vi "SampleApplication.vi"() -> ()   [LabVIEW 2009]
uses:
  TofDaqDll/TSharedMemoryDesc.ctl
  TofDaqDll/Dblx16.ctl
  TofDaqDll/charX256.ctl
  TofDaqDll/charX128.ctl
panel:
  in  "TSharedMemoryDesc":T1
  out "TofDaq running":bool
  out "peak mass":sgl
  out "peak label":string
  in  "peak index":i32
  out "profile":T5(graph)
  out "Mass Spec Axis Label":string
  in  "stop":bool
  in  "Stop":bool
  in  "Start":bool
  out "DAQ active":bool
  out "Mass spectra":T6(graph)
  in  "Axis type":i32=1
  in  "Normalize":bool=TRUE
  in  "SegmentIndex":i32 min=0 max=9 step=1
  out "error out":errorcluster
  in  "error in (no error)":errorcluster
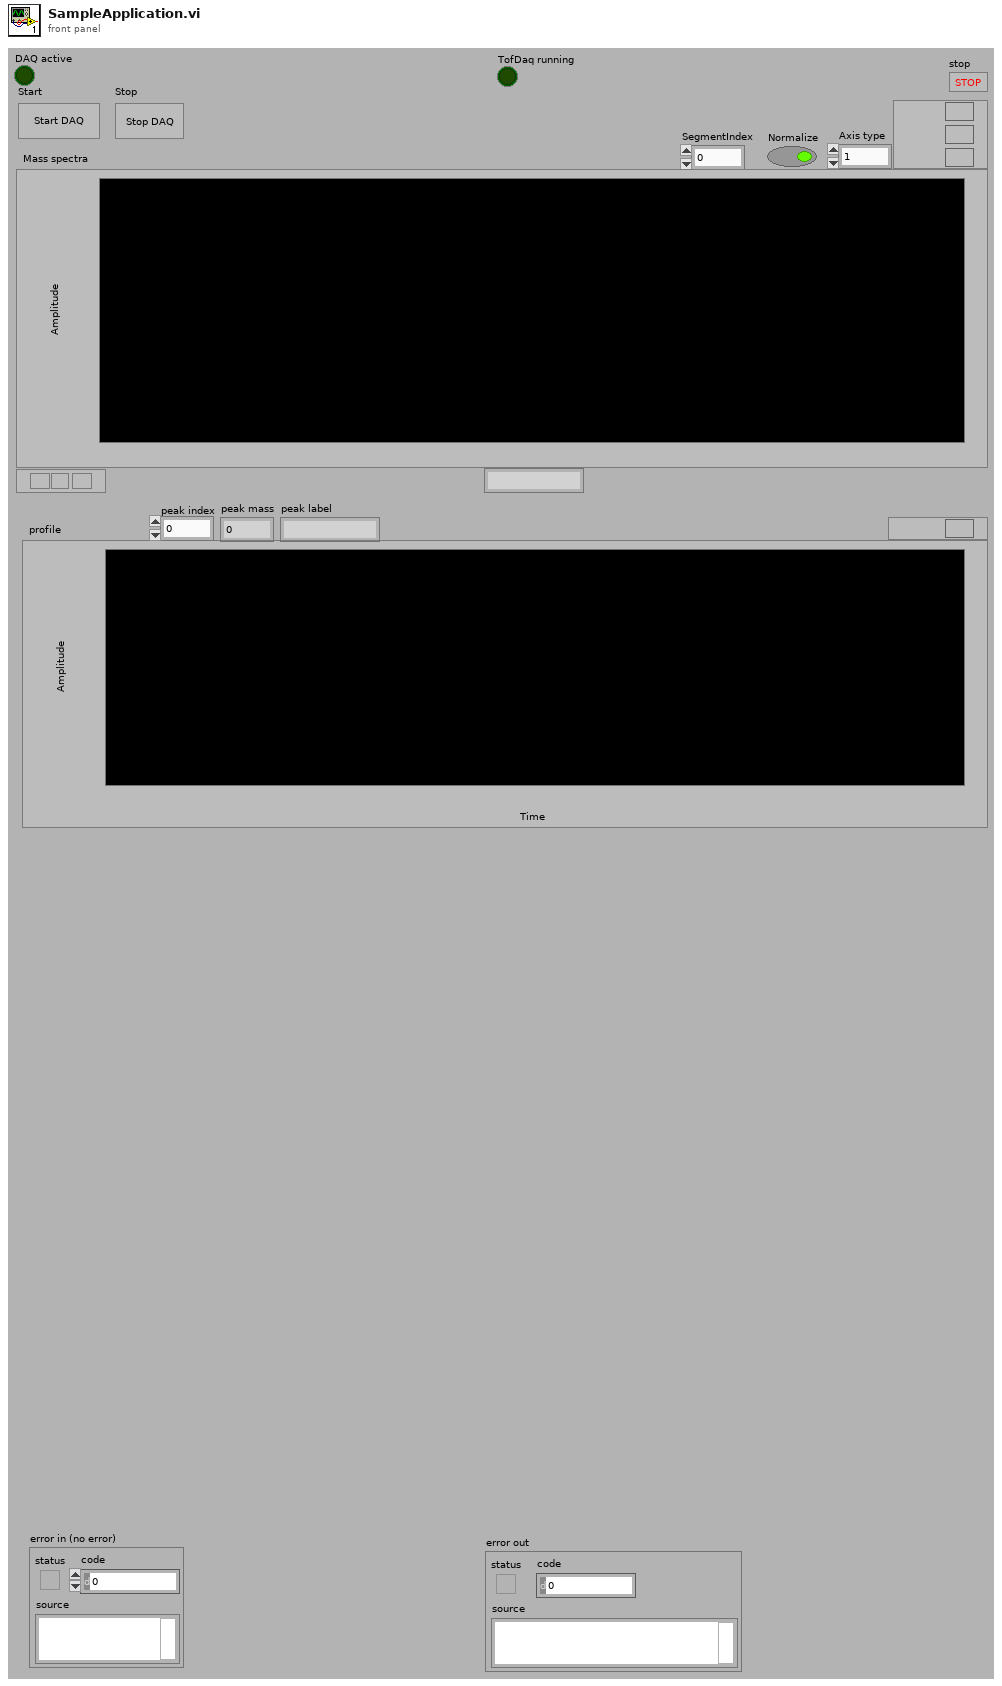
[diagram p1: front panel]
types:
  T1 = typedef "TSharedMemoryDesc.ctl" = cluster{"NbrSamples":i32, "NbrRawSamples":i32, "NbrPeaks":i32, "NbrWaveforms":i32, "NbrSegments":i32, "NbrBlocks":i32, "NbrMemories":i32, "NbrBufs":i32, "NbrWrites":i32, "NbrRuns":i32, "iWaveform":i32, "iSegment":i32, "iBlock":i32, "iMemory":i32, "iBuf":i32, "iWrite":i32, "iRun":i32, "TotalBufsRecorded":i32, "TotalBufsProcessed":i32, "TotalBufsWritten":i32, "OverallBufsProcessed":i32, "TotalNbrMemories":i32, "TotalMemoriesProcessed":i32, "RawDataRecordedBuf1":u32, "RawDataRecordedBuf2":u32, " RawDataLastElementInBuffer1 ":u32, " RawDataLastElementInBuffer2":u32, "RawDataProcessedBuf1":u32, "RawDataProcessedBuf2":u32, "RawDataWrittenBuf1":u32, "RawDataWrittenBuf2":u32, "SampleInterval":sgl, "TofPeriod":i32, "dummy":i32, "BlockPeriod":i64, "BlockPulseDelay":i64, " BlockDelay ":i64, "SingleIonSignal":sgl, "SingleIonSignal2":sgl, "MassCalibMode":i32, "MassCalibMode2":i32, "NbrMassCalibParams":i32, "NbrMassCalibParams2":i32, "p":T2, "p2":T2, "R0":sgl, "dm":sgl, "m0":sgl, "secondTof":u8, "chIniFileName":T3, "CurrentDataFileName":T3, "dummy":i8, "dummy 2":i8, "dummy 3":i8, "DaqMode":i32, " AcquisitionMode ":i32, "CombineMode":i32, "RecalibFreq":i32, "AcquisitionLogText":T3, " AcquisitionLogTime ":u64, "TimeZero":u64, "ExternalLock":u32, "ProcessingLevel":u32, "AttributeType":i32, "AttributeObject":T3, "AttributeName":T4, " AttributeInt ":i32, " AttributeDouble ":dbl, "EnableVarNbrMemories":u8, "dummy 4":i8, "dummy 5":i8, "dummy 6":i8, " NbrSteps":i32, "  CurrentStepAtBuf ":i32, "NbrMemoriesForCurrentStep":i32}
  T2 = typedef "Dblx16.ctl" = cluster{"0":dbl, "1":dbl, "2":dbl, "3":dbl, "4":dbl, "5":dbl, "6":dbl, "7":dbl, "8":dbl, "9":dbl, "10":dbl, "11":dbl, "12":dbl, "13":dbl, "14":dbl, "15":dbl}
  T3 = typedef "charX256.ctl" = cluster{i8, i8, i8, i8, i8, i8, i8, i8, i8, i8, i8, i8, i8, i8, i8, i8, i8, i8, i8, i8, i8, i8, i8, i8, i8, i8, i8, i8, i8, i8, i8, i8, i8, i8, i8, i8, i8, i8, i8, i8, i8, i8, i8, i8, i8, i8, i8, i8, i8, i8, i8, i8, i8, i8, i8, i8, i8, i8, i8, i8, i8, i8, i8, i8, i8, i8, i8, i8, i8, i8, i8, i8, i8, i8, i8, i8, i8, i8, i8, i8, i8, i8, i8, i8, i8, i8, i8, i8, i8, i8, i8, i8, i8, i8, i8, i8, i8, i8, i8, i8, i8, i8, i8, i8, i8, i8, i8, i8, i8, i8, i8, i8, i8, i8, i8, i8, i8, i8, i8, i8, i8, i8, i8, i8, i8, i8, i8, i8, i8, i8, i8, i8, i8, i8, i8, i8, i8, i8, i8, i8, i8, i8, i8, i8, i8, i8, i8, i8, i8, i8, i8, i8, i8, i8, i8, i8, i8, i8, i8, i8, i8, i8, i8, i8, i8, i8, i8, i8, i8, i8, i8, i8, i8, i8, i8, i8, i8, i8, i8, i8, i8, i8, i8, i8, i8, i8, i8, i8, i8, i8, i8, i8, i8, i8, i8, i8, i8, i8, i8, i8, i8, i8, i8, i8, i8, i8, i8, i8, i8, i8, i8, i8, i8, i8, i8, i8, i8, i8, i8, i8, i8, i8, i8, i8, i8, i8, i8, i8, i8, i8, i8, i8, i8, i8, i8, i8, i8, i8, i8, i8, i8, i8, i8, i8, i8, i8, i8, i8, i8, i8, i8, i8, i8, i8, i8, i8}
  T4 = typedef "charX128.ctl" = cluster{i8, i8, i8, i8, i8, i8, i8, i8, i8, i8, i8, i8, i8, i8, i8, i8, i8, i8, i8, i8, i8, i8, i8, i8, i8, i8, i8, i8, i8, i8, i8, i8, i8, i8, i8, i8, i8, i8, i8, i8, i8, i8, i8, i8, i8, i8, i8, i8, i8, i8, i8, i8, i8, i8, i8, i8, i8, i8, i8, i8, i8, i8, i8, i8, i8, i8, i8, i8, i8, i8, i8, i8, i8, i8, i8, i8, i8, i8, i8, i8, i8, i8, i8, i8, i8, i8, i8, i8, i8, i8, i8, i8, i8, i8, i8, i8, i8, i8, i8, i8, i8, i8, i8, i8, i8, i8, i8, i8, i8, i8, i8, i8, i8, i8, i8, i8, i8, i8, i8, i8, i8, i8, i8, i8, i8, i8, i8, i8}
  T5 = cluster{"profile time":dbl[], "profile data":sgl[]}
  T6 = cluster{"SpecAxis out":dbl[], "SumSpectrum out":dbl[]}[]
  T7 = cluster{"label":string, "mass":sgl, "loMass":sgl, "hiMass":sgl}
  T8 = cluster{"SpecAxis out":dbl[], "Tof spectrum out":sgl[]}
  T9 = cluster{"Masses out":sgl[], "Stick spectrum out":sgl[]}
  T10 = cluster{"SpecAxis out":dbl[], "SumSpectrum out":dbl[]}
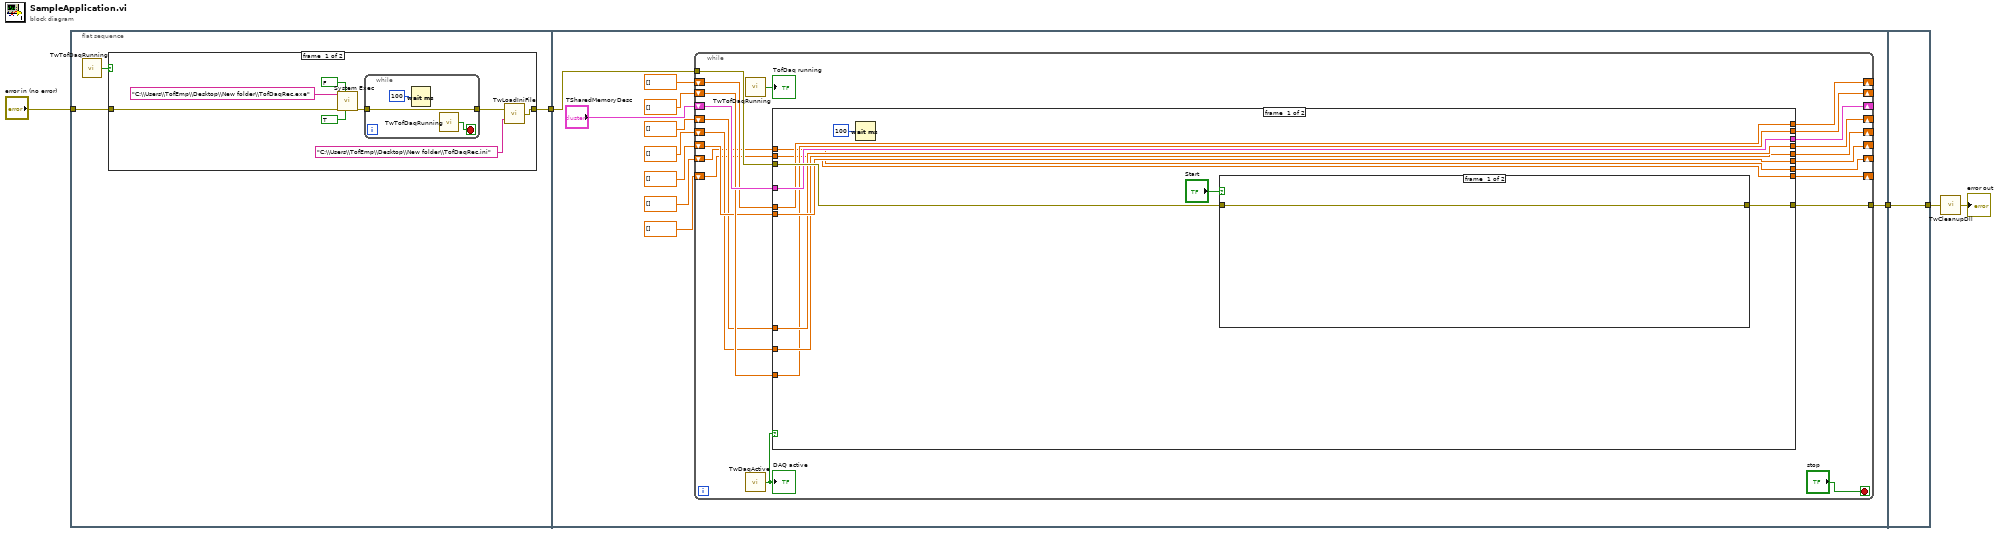
[diagram p0: block diagram]
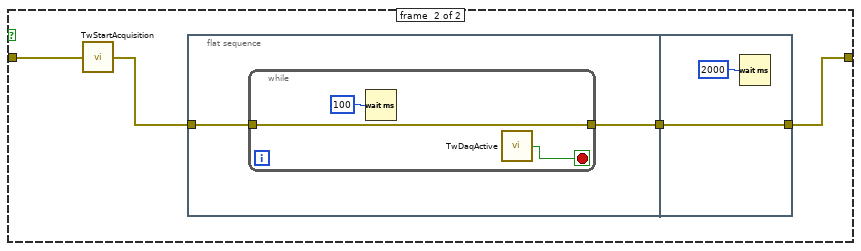
[diagram p3: hidden frame]
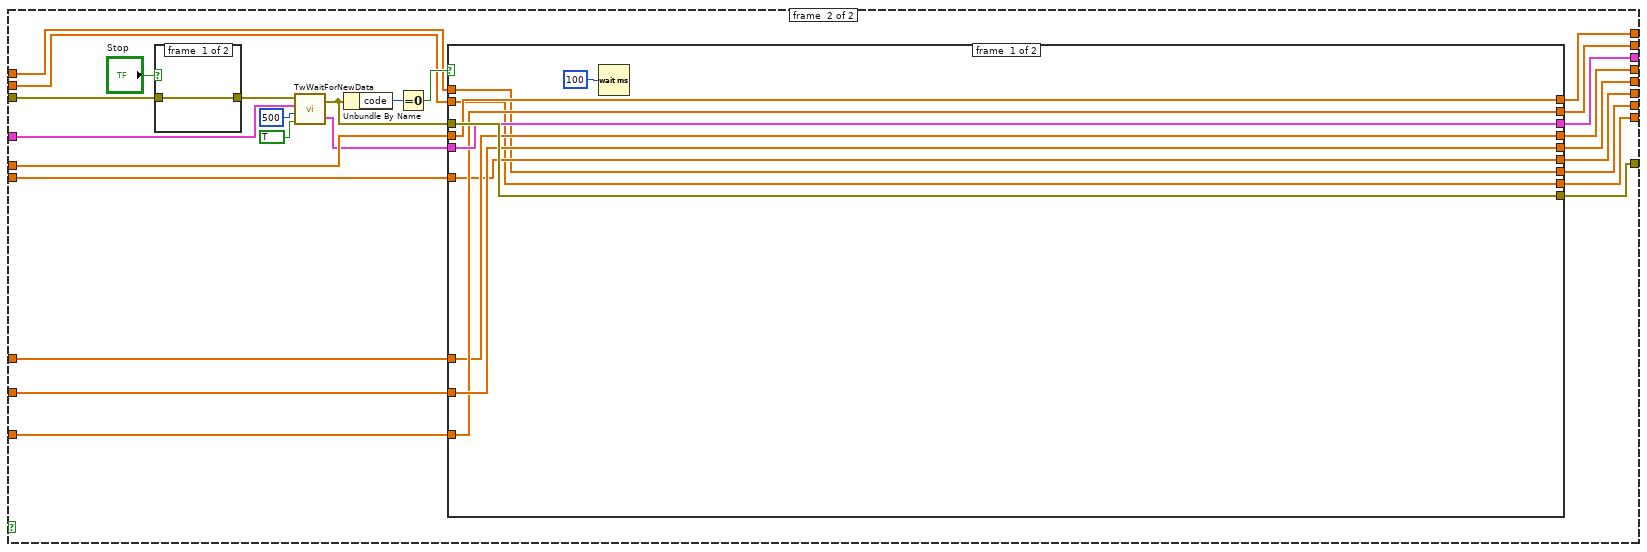
[diagram p4: hidden frame]
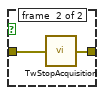
[diagram p5: hidden frame]
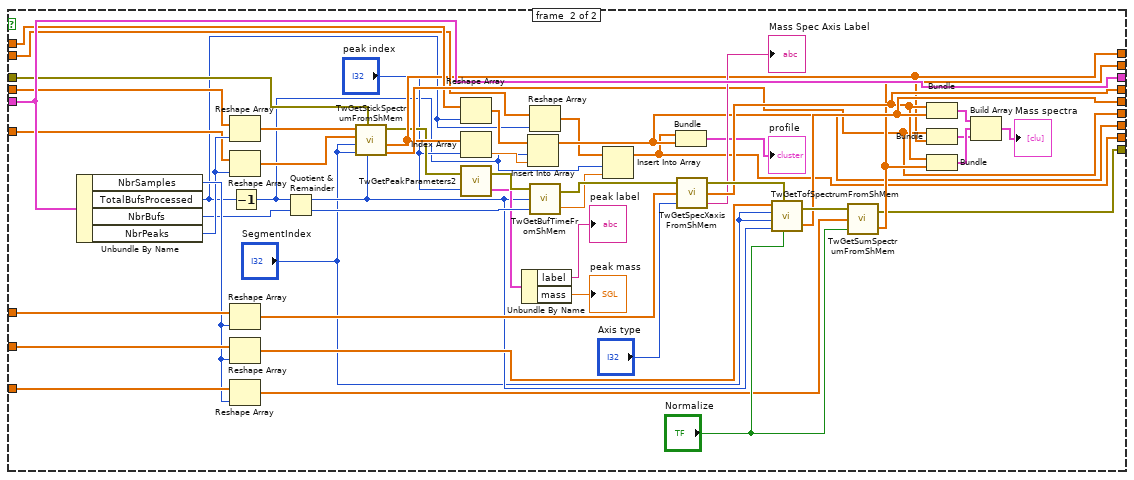
[diagram p6: hidden frame]
diagram:
  n1 = flat-sequence {
    tunnel: "error in (no error)" -> [w7]
    tunnel: [w6] -> w5
    tunnel: w5 -> [w30]
    tunnel: [w22] -> w4
    tunnel: [w166] -> w3
    tunnel: w4 -> [w166]
    frame #0 {
      n2 = call "TwTofDaqRunning.vi"() -> ("running?"=w8:bool)
      n3 = case shown="False" w8 {
        tunnel: w7 -> [w16 w20]
        tunnel: [w10 w20] -> w6
        frame #0 {
          n4 = call <vilib>:"System Exec.vi"("run minimized? (F)"=TRUE, "wait until completion? (T)"=FALSE, "error in (no error)"=w16, "command line"="C:\\Users\\TofEmp\\Desktop\\New folder\\TofDaqRec.exe") -> ("error out"=w12:errorcluster)  [unwired: 2 in, 5 out]
          n5 = while {
            tunnel: [w17] -> w11
            tunnel: w12 -> [w17]
            stop <- w19 stop-if-true
            n6 = Wait (ms)(milliseconds to wait=u32 100) -> ()  [unwired: 1 out]
            n7 = call "TwTofDaqRunning.vi"() -> ("running?"=w19:bool)
          }
          n8 = call "TwLoadIniFile.vi"("IniFile"="C:\\Users\\TofEmp\\Desktop\\New folder\\TofDaqRec.ini", "error in (no error)"=w11) -> ("error out"=w10:errorcluster)
        }
        frame #1 {
        }
      }
    }
    frame #1 {
      n9 = while {
        tunnel: w30 -> [w51]
        tunnel: [w48] -> w22
        shift-right: [w32] -> _
        shift-left: "TSharedMemoryDesc" -> [w43]
        shift-right: [w37] -> _
        shift-left: sgl[] [] ("Stick spectrum in") -> [w42]
        shift-right: [w44] -> _
        shift-left: sgl[] [] ("Masses in") -> [w40]
        shift-right: [w45] -> _
        shift-left: dbl[] [] ("SpecAxis in") -> [w39]
        shift-right: [w46] -> _
        shift-left: sgl[] [] ("Tof spectrum") -> [w38]
        shift-right: [w47] -> _
        shift-left: dbl[] [] ("SumSpectrum in") -> [w41]
        shift-right: [w34] -> _
        shift-left: sgl[] [] ("profile data") -> [w36]
        shift-right: [w35] -> _
        shift-left: dbl[] [] ("profile time") -> [w33]
        stop <- "stop" stop-if-true
        n10 = call "TwTofDaqRunning.vi"() -> ("running?"=→"TofDaq running":bool)
        n11 = call "TwDaqActive.vi"() -> ("DAQ active?"=w50:bool)
        "DAQ active" <- w50
        n12 = case shown="True" w50 {
          tunnel: w51 -> [w61 w94]
          tunnel: [w60 w100] -> w48
          tunnel: [w54 w92] -> w47
          tunnel: [w55 w91] -> w46
          tunnel: [w56 w90] -> w45
          tunnel: [w58 w89] -> w37
          tunnel: [w59 w88] -> w32
          tunnel: [w57 w87] -> w44
          tunnel: w43 -> [w59 w77]
          tunnel: w42 -> [w58 w86]
          tunnel: w41 -> [w54 w85]
          tunnel: w40 -> [w57 w84]
          tunnel: w39 -> [w56 w83]
          tunnel: w38 -> [w55 w82]
          tunnel: w36 -> [w53 w81]
          tunnel: w33 -> [w52 w80]
          tunnel: [w53 w79] -> w34
          tunnel: [w52 w78] -> w35
          frame #0 {
            n13 = Wait (ms)(milliseconds to wait=u32 100) -> ()  [unwired: 1 out]
            n14 = case shown="False" "Start" {
              tunnel: w61 -> [w64 w68]
              tunnel: [w64 w66] -> w60
              frame #0 {
              }
              frame #1 {
                n15 = call "TwStartAcquisition.vi"("error in (no error)"=w68) -> ("error out"=w67:errorcluster)
                n16 = flat-sequence {
                  tunnel: w67 -> [w70]
                  tunnel: [w69] -> w65
                  tunnel: [w75] -> w66
                  tunnel: w65 -> [w75]
                  frame #0 {
                    n17 = while {
                      tunnel: [w72] -> w69
                      tunnel: w70 -> [w72]
                      stop <- w71 stop-if-true
                      n18 = Wait (ms)(milliseconds to wait=u32 100) -> ()  [unwired: 1 out]
                      n19 = call "TwDaqActive.vi"() -> ("DAQ active?"=w71:bool)
                    }
                  }
                  frame #1 {
                    n20 = Wait (ms)(milliseconds to wait=u32 2000) -> ()  [unwired: 1 out]
                  }
                }
              }
            }
          }
          frame #1 {
            n21 = case shown="False" "Stop" {
              tunnel: w94 -> [w102 w104]
              tunnel: [w102 w103] -> w93
              frame #0 {
              }
              frame #1 {
                n22 = call "TwStopAcquisition.vi"("error in (no error)"=w104) -> ("error out"=w103:errorcluster)
              }
            }
            n23 = call "TwWaitForNewData.vi"("WaitForEventReset"=TRUE, "Timeout"=500, "TSharedMemoryDesc in"=w77, "error in (no error)"=w93) -> ("TSharedMemoryDesc out"=w76:T1, "error out"=w99:errorcluster)
            n24 = Unbundle By Name(w99) -> ("code"=w98:i32)
            n25 = Equal To 0?(x=w98) -> (x = 0?=w97:bool)
            n26 = case shown="True" w97 {
              tunnel: [w114 w139] -> w100
              tunnel: w99 -> [w114 w138]
              tunnel: w76 -> [w113 w163]
              tunnel: [w113 w163] -> w88
              tunnel: w82 -> [w111 w165]
              tunnel: [w111 w153] -> w91
              tunnel: w85 -> [w110 w160]
              tunnel: [w110 w150] -> w92
              tunnel: w83 -> [w109 w157]
              tunnel: [w109 w151] -> w90
              tunnel: [w108 w126] -> w89
              tunnel: [w107 w141] -> w87
              tunnel: w86 -> [w108 w146]
              tunnel: w84 -> [w107 w143]
              tunnel: w81 -> [w106 w133]
              tunnel: w80 -> [w105 w132]
              tunnel: [w106 w136] -> w79
              tunnel: [w105 w135] -> w78
              frame #0 {
                n27 = Wait (ms)(milliseconds to wait=u32 100) -> ()  [unwired: 1 out]
              }
              frame #1 {
                n28 = Unbundle By Name(w163) -> ("NbrSamples"=w155:i32, "TotalBufsProcessed"=w124:i32, "NbrBufs"=w137:i32, "NbrPeaks"=w144:i32)
                n29 = Reshape Array(w146, w144) -> (w145:sgl[])
                n30 = Reshape Array(w143, w144) -> (w142:sgl[])
                n31 = Reshape Array(w157, w155) -> (w156:dbl[])
                n32 = Reshape Array(w165, w155) -> (w164:sgl[])
                n33 = Reshape Array(w160, w155) -> (w159:dbl[])
                n34 = Decrement(x=w124) -> (x-1=w117:i32)
                n35 = Quotient & Remainder(x=w117, y=w137) -> (x-y*floor(x/y)=w116:i32, floor(x/y)=w129:i32)
                n36 = call "TwGetStickSpectrumFromShMem.vi"("BufIndex"=w116, "error in (no error)"=w138, "SegmentEndIndex"="SegmentIndex", "SegmentIndex"="SegmentIndex", "Masses in"=w142, "Stick spectrum in"=w145) -> ("Masses out"=w141:sgl[], "Stick spectrum out"=w126:sgl[], "error out"=w123:errorcluster)  [unwired: 1 in]
                n37 = Reshape Array(w133, w124) -> (w131:sgl[])
                n38 = Index Array(array=w126, index="peak index") -> (element=w125:sgl)
                n39 = call "TwGetPeakParameters2.vi"("PeakIndex"="peak index", "error in (no error)"=w123) -> ("PeakPar out"=w120:T7, "error out"=w122:errorcluster)
                n40 = Unbundle By Name(w120) -> ("label"=→"peak label":string, "mass"=→"peak mass":sgl)
                n41 = Insert Into Array(array=w131, index=w117, new element=w125) -> (w136:sgl[])
                n42 = Reshape Array(w132, w124) -> (w130:dbl[])
                n43 = call "TwGetBufTimeFromShMem.vi"("WriteIndex"=w129, "BufIndex"=w116, "error in (no error)"=w122) -> ("BufTime"=w127:dbl, "error out"=w128:errorcluster)
                n44 = Insert Into Array(array=w130, index=w117, new element=w127) -> (w135:dbl[])
                n45 = Bundle("profile time"=w135, "profile data"=w136) -> (→"profile":T5)  [unwired: 1 out]
                n46 = call "TwGetSpecXaxisFromShMem.vi"("Axis type"="Axis type", "SpecAxis in"=w156, "error in (no error)"=w128) -> ("UnitLabel"=→"Mass Spec Axis Label":string, "SpecAxis out"=w151:dbl[], "error out"=w158:errorcluster)
                n47 = call "TwGetTofSpectrumFromShMem.vi"("Normalize"="Normalize", "error in (no error)"=w158, "BufIndex"=w116, "SegmentEndIndex"="SegmentIndex", "SegmentIndex"="SegmentIndex", "Tof spectrum in"=w164) -> ("Tof spectrum out"=w153:sgl[], "error out"=w162:errorcluster)
                n48 = call "TwGetSumSpectrumFromShMem.vi"("Normalize"="Normalize", "SumSpectrum in"=w159, "error in (no error)"=w162) -> ("SumSpectrum out"=w150:dbl[], "error out"=w139:errorcluster)
                n49 = Bundle("SpecAxis out"=w151, "Tof spectrum out"=w153) -> (w152:T8)  [unwired: 1 out]
                n50 = Bundle("Masses out"=w141, "Stick spectrum out"=w126) -> (w140:T9)  [unwired: 1 out]
                n51 = Bundle("SpecAxis out"=w151, "SumSpectrum out"=w150) -> (w149:T10)  [unwired: 1 out]
                n52 = Build Array(w152, w149, w140) -> (→"Mass spectra":T6)
              }
            }
          }
        }
      }
    }
    frame #2 {
    }
  }
  n53 = call "TwCleanupDll.vi"("error in (no error)"=w3) -> ("error out"=→"error out":errorcluster)
